vi "Populate Scope.vi"(8 "Error In":errorcluster, 11 "State In":T1) -> (0 "Error Out":errorcluster, 3 "State Out":T1)   [LabVIEW 2017, in "Eulogy.lvlib" / "Bookmark Manager.lvlib"]
uses:
  Bookmark Manager.lvlib
  State.ctl
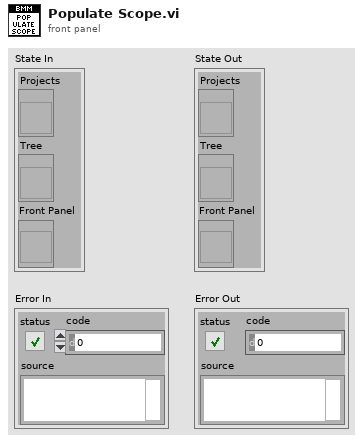
[diagram p1: front panel]
types:
  T1 = typedef "Eulogy.lvlib/Bookmark Manager.lvlib/State.ctl" = cluster{"Projects":refnum<vi>, "Tree":refnum<vi>, "Front Panel":refnum<vi>}
  T2 = enum8{"Enabled", "Disabled", "Disabled and Grayed Out"}
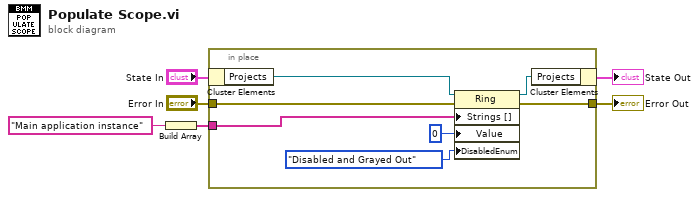
[diagram p0: block diagram]
diagram:
  n1 = Build Array("Main application instance") -> (w5:string[])
  n2 = in-place {
    in-place-border: w5 -> [w11]
    in-place-border: "Error In" -> [w8]
    in-place-border: [w7] -> w3
    n3 = in-place-cluster #1("State In") -> ("Projects"=w13:refnum<vi>)
    n4 = property class="Ring"(reference=w13, error in=w8, "Strings []"=w11, "Value"=u16 0, "DisabledEnum"=T2."Disabled and Grayed Out" ("Disabled")) -> (reference out=w12:refnum<vi>, error out=w7:errorcluster)
    n5 = in-place-cluster #1("Projects"=w12) -> (→"State Out":T1)
  }
  "Error Out" <- w3
